vi "Hot Goal Recognition.vi"() -> (0 "Right Goal Hot?":bool, 1 "Left Goal hot?":bool)   [LabVIEW 2013]
uses:
  <vilib>/Rock Robotics/WPI/Camera/WPI_CameraSettings Read MJPG.ctl
  <vilib>/Rock Robotics/WPI/Camera/WPI_CameraImageSize.ctl
  <vilib>/vision/NI_Vision_Development_Module.lvlib
panel:
  out "ERROR":bool
  out "Image":T1(plugin-control)
  out "error out":errorcluster
  in  "Camera IP":string="10.9.0.11"
  out "Bandwidth (Mbps)":dbl
  in  "Camera Settings":T2={"fps"=30, "compression"=30, "Image Size"=enum."320x240"}
  # "do not change resolution!!!! (320x240)"
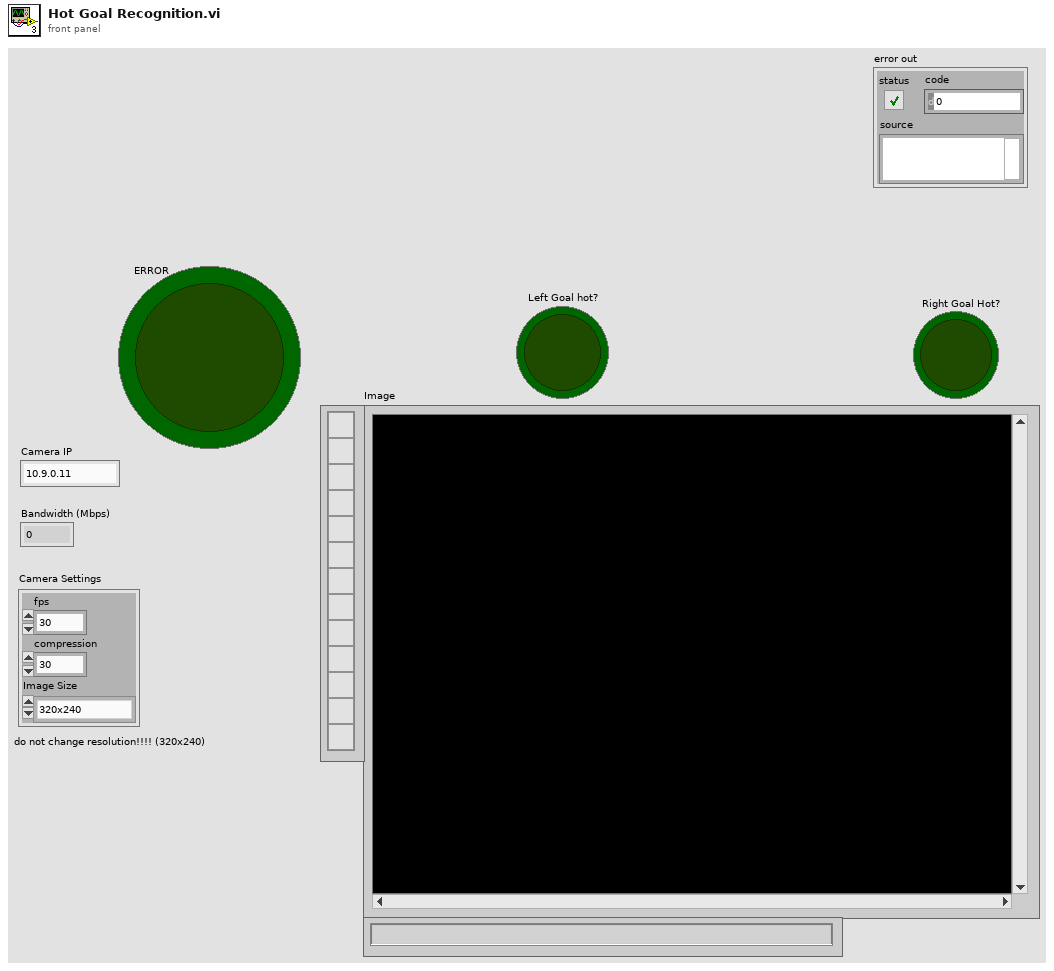
[diagram p1: front panel]
types:
  T1 = typedef "IMAQ Image.ctl" = refnum<image>
  T2 = typedef "WPI_CameraSettings Read MJPG.ctl" = cluster{"fps":i32, "compression":i32, "Image Size":T3}
  T3 = typedef "WPI_CameraImageSize.ctl" = enum16{"640x480", "320x240", "160x120"}
  T4 = typedef "Image Type" = u32
  T5 = enum32{"AutoM", "Close", "Dilate", "Erode", "Gradient", "Gradient in", "Gradient out", "HitMiss", "Open", "PClose", "POpen", "Thick", "Thin"}
  T6 = typedef "Particle Parameters" = i32
  T7 = cluster{"Particle Measurements (Pixels)[0]":dbl, "Particle Measurements (Pixels)[1]":dbl}
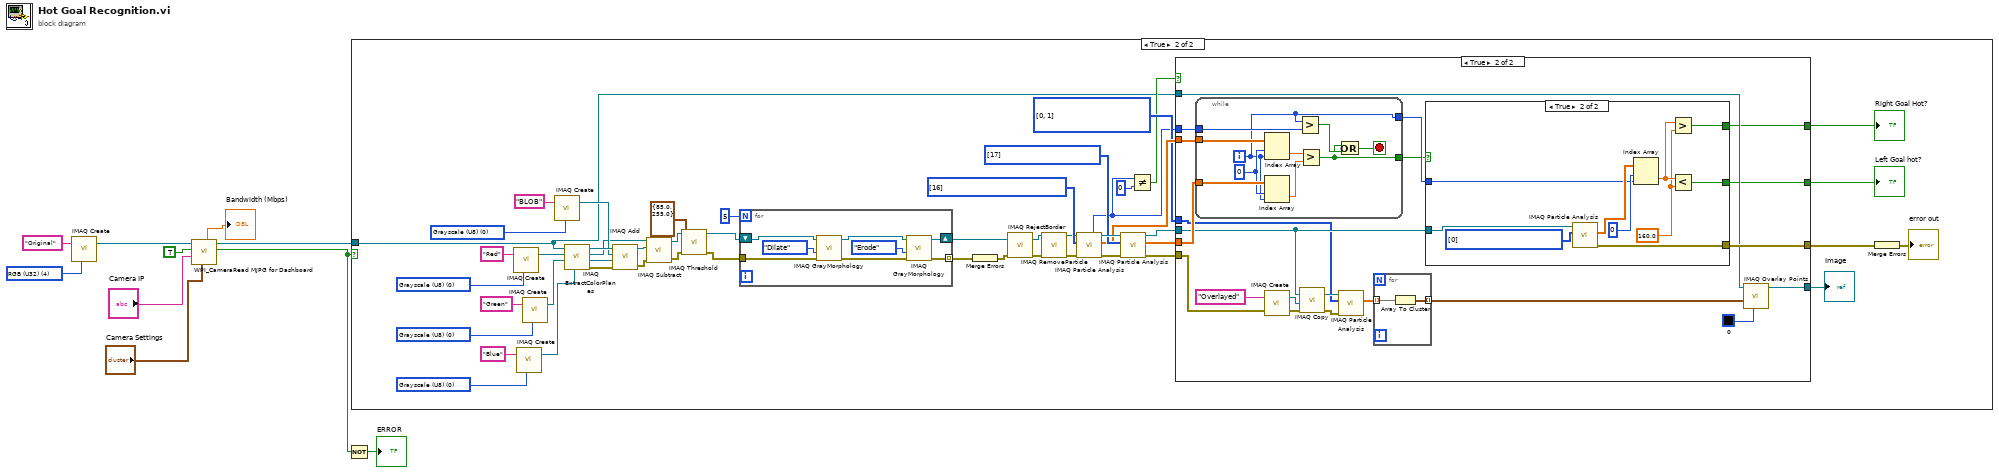
[diagram p0: block diagram]
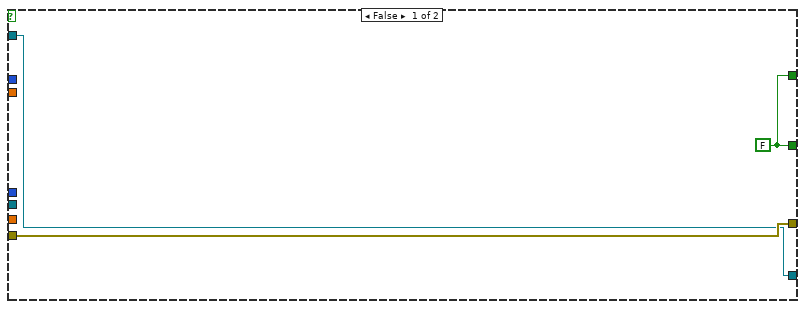
[diagram p3: hidden frame]
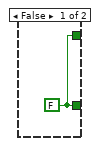
[diagram p4: hidden frame]
diagram:
  w1 = T4 4 items=["Grayscale (U8)", "Grayscale (I16)", "Grayscale (SGL)", "Complex (CSG)", "RGB (U32)", "HSL (U32)", "RGB (U64)", "Grayscale (U16)"] ("Image Type")
  n1 = call "IMAQ Create"("Image Name"="Original", "Image Type"=w1) -> ("New Image"=w9:T1)  [unwired: 3 in, 1 out]
  n2 = call <vilib>:"WPI_CameraRead MJPG for Dashboard.vi"("Camera Settings"="Camera Settings", "Camera IP"="Camera IP", "Enable"=TRUE, "Refnum in"=w9) -> ("Active"=w6:bool, "Refnum out"=w7:T1, "Bandwidth (Mbps)"=→"Bandwidth (Mbps)":dbl)  [unwired: 4 in, 1 out]
  n3 = Not(x=w6) -> (.not. x?=→"ERROR":bool)
  n4 = case shown="True" w6 {
    tunnel: w7 -> [_ w21]
    frame False {
    }
    frame True {
      w26 = T6[] [0, 1] items=["Center of Mass X", "Center of Mass Y", "First Pixel X", "First Pixel Y", "Bounding Rect Left", "Bounding Rect Top", "Bounding Rect Right", "Bounding Rect Bottom", "Max Feret Diameter Start X", "Max Feret Diameter Start Y", "Max Feret Diameter End X", "Max Feret Diameter End Y", "Max Horiz. Segment Length Left", "Max Horiz. Segment Length Right", "Max Horiz. Segment Length Row", "-", "Bounding Rect Width", "Bounding Rect Height", "Bounding Rect Diagonal", "Perimeter", "Convex Hull Perimeter", "Holes' Perimeter", "Max Feret Diameter", "Equivalent Ellipse Major Axis", "Equivalent Ellipse Minor Axis", "Equivalent Ellipse Minor Axis (Feret)", "Equivalent Rect Long Side", "Equivalent Rect Short Side", "Equivalent Rect Diagonal", "Equivalent Rect Short Side (Feret)", "Average Horiz. Segment Length", "Average Vert. Segment Length", "Hydraulic Radius", "Waddel Disk Diameter", "-", "Area", "Holes' Area", "Particle & Holes' Area", "Convex Hull Area", "Image Area", "-", "Number of Holes", "Number of Horiz. Segments", "Number of Vert. Segments", "-", "Orientation", "Max Feret Diameter Orientation", "-", "% Area/Image Area", "% Area/(Particle & Holes' Area)", "Ratio of Equivalent Ellipse Axes", "Ratio of Equivalent Rect Sides", "-", "Elongation Factor", "Compactness Factor", "Heywood Circularity Factor", "Type Factor", "-", "Sum X", "Sum Y", "Sum XX", "Sum XY", "Sum YY", "Sum XXX", "Sum XXY", "Sum XYY", "Sum YYY", "-", "Moment of Inertia XX", "Moment of Inertia XY", "Moment of Inertia YY", "Moment of Inertia XXX", "Moment of Inertia XXY", "Moment of Inertia XYY", "Moment of Inertia YYY", "Norm. Moment of Inertia XX", "Norm. Moment of Inertia XY", "Norm. Moment of Inertia YY", "Norm. Moment of Inertia XXX", "Norm. Moment of Inertia XXY", "Norm. Moment of Inertia XYY", "Norm. Moment of Inertia YYY", "Hu Moment 1", "Hu Moment 2", "Hu Moment 3", "Hu Moment 4", "Hu Moment 5", "Hu Moment 6", "Hu Moment 7"] ("Pixel Measurements")
      w45 = T4 0 items=["Grayscale (U8)", "Grayscale (I16)", "Grayscale (SGL)", "Complex (CSG)", "RGB (U32)", "HSL (U32)", "RGB (U64)", "Grayscale (U16)"] ("Image Type")
      w48 = T4 0 items=["Grayscale (U8)", "Grayscale (I16)", "Grayscale (SGL)", "Complex (CSG)", "RGB (U32)", "HSL (U32)", "RGB (U64)", "Grayscale (U16)"] ("Image Type")
      w50 = T4 0 items=["Grayscale (U8)", "Grayscale (I16)", "Grayscale (SGL)", "Complex (CSG)", "RGB (U32)", "HSL (U32)", "RGB (U64)", "Grayscale (U16)"] ("Image Type")
      w55 = T6[] [17] items=["Center of Mass X", "Center of Mass Y", "First Pixel X", "First Pixel Y", "Bounding Rect Left", "Bounding Rect Top", "Bounding Rect Right", "Bounding Rect Bottom", "Max Feret Diameter Start X", "Max Feret Diameter Start Y", "Max Feret Diameter End X", "Max Feret Diameter End Y", "Max Horiz. Segment Length Left", "Max Horiz. Segment Length Right", "Max Horiz. Segment Length Row", "-", "Bounding Rect Width", "Bounding Rect Height", "Bounding Rect Diagonal", "Perimeter", "Convex Hull Perimeter", "Holes' Perimeter", "Max Feret Diameter", "Equivalent Ellipse Major Axis", "Equivalent Ellipse Minor Axis", "Equivalent Ellipse Minor Axis (Feret)", "Equivalent Rect Long Side", "Equivalent Rect Short Side", "Equivalent Rect Diagonal", "Equivalent Rect Short Side (Feret)", "Average Horiz. Segment Length", "Average Vert. Segment Length", "Hydraulic Radius", "Waddel Disk Diameter", "-", "Area", "Holes' Area", "Particle & Holes' Area", "Convex Hull Area", "Image Area", "-", "Number of Holes", "Number of Horiz. Segments", "Number of Vert. Segments", "-", "Orientation", "Max Feret Diameter Orientation", "-", "% Area/Image Area", "% Area/(Particle & Holes' Area)", "Ratio of Equivalent Ellipse Axes", "Ratio of Equivalent Rect Sides", "-", "Elongation Factor", "Compactness Factor", "Heywood Circularity Factor", "Type Factor", "-", "Sum X", "Sum Y", "Sum XX", "Sum XY", "Sum YY", "Sum XXX", "Sum XXY", "Sum XYY", "Sum YYY", "-", "Moment of Inertia XX", "Moment of Inertia XY", "Moment of Inertia YY", "Moment of Inertia XXX", "Moment of Inertia XXY", "Moment of Inertia XYY", "Moment of Inertia YYY", "Norm. Moment of Inertia XX", "Norm. Moment of Inertia XY", "Norm. Moment of Inertia YY", "Norm. Moment of Inertia XXX", "Norm. Moment of Inertia XXY", "Norm. Moment of Inertia XYY", "Norm. Moment of Inertia YYY", "Hu Moment 1", "Hu Moment 2", "Hu Moment 3", "Hu Moment 4", "Hu Moment 5", "Hu Moment 6", "Hu Moment 7"] ("Pixel Measurements")
      w57 = T6[] [16] items=["Center of Mass X", "Center of Mass Y", "First Pixel X", "First Pixel Y", "Bounding Rect Left", "Bounding Rect Top", "Bounding Rect Right", "Bounding Rect Bottom", "Max Feret Diameter Start X", "Max Feret Diameter Start Y", "Max Feret Diameter End X", "Max Feret Diameter End Y", "Max Horiz. Segment Length Left", "Max Horiz. Segment Length Right", "Max Horiz. Segment Length Row", "-", "Bounding Rect Width", "Bounding Rect Height", "Bounding Rect Diagonal", "Perimeter", "Convex Hull Perimeter", "Holes' Perimeter", "Max Feret Diameter", "Equivalent Ellipse Major Axis", "Equivalent Ellipse Minor Axis", "Equivalent Ellipse Minor Axis (Feret)", "Equivalent Rect Long Side", "Equivalent Rect Short Side", "Equivalent Rect Diagonal", "Equivalent Rect Short Side (Feret)", "Average Horiz. Segment Length", "Average Vert. Segment Length", "Hydraulic Radius", "Waddel Disk Diameter", "-", "Area", "Holes' Area", "Particle & Holes' Area", "Convex Hull Area", "Image Area", "-", "Number of Holes", "Number of Horiz. Segments", "Number of Vert. Segments", "-", "Orientation", "Max Feret Diameter Orientation", "-", "% Area/Image Area", "% Area/(Particle & Holes' Area)", "Ratio of Equivalent Ellipse Axes", "Ratio of Equivalent Rect Sides", "-", "Elongation Factor", "Compactness Factor", "Heywood Circularity Factor", "Type Factor", "-", "Sum X", "Sum Y", "Sum XX", "Sum XY", "Sum YY", "Sum XXX", "Sum XXY", "Sum XYY", "Sum YYY", "-", "Moment of Inertia XX", "Moment of Inertia XY", "Moment of Inertia YY", "Moment of Inertia XXX", "Moment of Inertia XXY", "Moment of Inertia XYY", "Moment of Inertia YYY", "Norm. Moment of Inertia XX", "Norm. Moment of Inertia XY", "Norm. Moment of Inertia YY", "Norm. Moment of Inertia XXX", "Norm. Moment of Inertia XXY", "Norm. Moment of Inertia XYY", "Norm. Moment of Inertia YYY", "Hu Moment 1", "Hu Moment 2", "Hu Moment 3", "Hu Moment 4", "Hu Moment 5", "Hu Moment 6", "Hu Moment 7"] ("Pixel Measurements")
      w58 = T4 0 items=["Grayscale (U8)", "Grayscale (I16)", "Grayscale (SGL)", "Complex (CSG)", "RGB (U32)", "HSL (U32)", "RGB (U64)", "Grayscale (U16)"] ("Image Type")
      n5 = call "IMAQ Create"("Image Name"="Red", "Image Type"=w50) -> ("New Image"=w51:T1)  [unwired: 3 in, 1 out]
      n6 = call "IMAQ Create"("Image Name"="Blue", "Image Type"=w45) -> ("New Image"=w44:T1)  [unwired: 3 in, 1 out]
      n7 = call "IMAQ Create"("Image Name"="Green", "Image Type"=w48) -> ("New Image"=w47:T1)  [unwired: 3 in, 1 out]
      n8 = call "IMAQ Create"("Image Name"="BLOB", "Image Type"=w58) -> ("New Image"=w41:T1)  [unwired: 3 in, 1 out]
      n9 = call "IMAQ ExtractColorPlanes"("Blue or Luma or Val or Inten Plane"=w44, "Green or Sat Plane"=w47, "Red or Hue Plane"=w51, "Image Src"=w21) -> ("error out"=w18:errorcluster, "Blue or Luma or Val or Inten Plane out"=w42:T1, "Green or Sat Plane out"=w40:T1, "Red or Hue Plane out"=w43:T1)  [unwired: 4 in]
      n10 = call "IMAQ Add"("Image Src A"=w43, "Image Dst"=w41, "Image Src B"=w42, "error in (no error)"=w18) -> ("Image Dst Out"=w17:T1, "error out"=w14:errorcluster)  [unwired: 3 in]
      n11 = call "IMAQ Subtract"("Image Src A"=w40, "Image Dst"=w17, "error in (no error)"=w14) -> ("Image Dst Out"=w15:T1, "error out"=w13:errorcluster)  [unwired: 4 in]
      n12 = call "IMAQ Threshold"("error in (no error)"=w13, "Range"=cluster{"Lower value":sgl, "Upper value":sgl} {"Lower value"=85.0, "Upper value"=255.0}, "Image Src"=w15) -> ("error out"=w12:errorcluster, "Image Dst Out"=w16:T1)  [unwired: 7 in]
      n13 = for {
        N: 5 -> [_]
        shift-right: [w110] -> w38
        shift-left: w16 -> [w111]
        tunnel: w12 -> [w109]
        tunnel: [w107] -> w35 mode=indexing
        n14 = call "IMAQ GrayMorphology"("error in (no error)"=w109, "Operation"=T5."Dilate", "Image Src"=w111) -> ("error out"=w108:errorcluster, "Image Dst Out"=w112:T1)  [unwired: 7 in]
        n15 = call "IMAQ GrayMorphology"("error in (no error)"=w108, "Operation"=T5."Erode", "Image Src"=w112) -> ("error out"=w107:errorcluster, "Image Dst Out"=w110:T1)  [unwired: 7 in]
      }
      n16 = Merge Errors(w35) -> (w34:errorcluster)
      n17 = call "IMAQ RejectBorder"("error in (no error)"=w34, "Image Src"=w38) -> ("error out"=w36:errorcluster, "Image Dst Out"=w37:T1)  [unwired: 4 in]
      n18 = call "IMAQ RemoveParticle"("error in (no error)"=w36, "Image Src"=w37) -> ("error out"=w29:errorcluster, "Image Dst Out"=w30:T1)  [unwired: 8 in]
      n19 = call "IMAQ Particle Analysis"("error in (no error)"=w29, "Pixel Measurements"=w57, "Image"=w30) -> ("error out"=w33:errorcluster, "Particle Measurements (Pixels)"=w54:dbl[][], "Image Out (duplicate)"=w56:T1, "Number of Particles"=w25:i32)  [unwired: 3 in, 2 out]
      n20 = call "IMAQ Particle Analysis"("error in (no error)"=w33, "Pixel Measurements"=w55, "Image"=w56) -> ("error out"=w27:errorcluster, "Particle Measurements (Pixels)"=w53:dbl[][], "Image Out (duplicate)"=w28:T1)  [unwired: 3 in, 3 out]
      n21 = Not Equal?(x=w25, y=0) -> (x != y?=w23:bool)
      n22 = case shown="True" w23 {
        tunnel: w54 -> [_ w83]
        tunnel: w53 -> [_ w82]
        tunnel: w25 -> [_ w81]
        tunnel: [w62 w78] -> w32
        tunnel: w28 -> [_ w75]
        tunnel: w27 -> [w62 w74]
        tunnel: w26 -> [_ w70]
        tunnel: [w61 w66] -> w22
        tunnel: w21 -> [w61 w65]
        tunnel: [w60 w64] -> w20
        tunnel: [w60 w63] -> w19
        frame False {
          w60 = FALSE
        }
        frame True {
          n23 = while {
            tunnel: w83 -> [w105]
            tunnel: w82 -> [w106]
            tunnel: w81 -> [w99]
            tunnel: [w98] -> w79
            tunnel: [w97] -> w80
            i -> [w97]
            stop <- w100 stop-if-true
            w104 = 0 ("disabled index (row)")
            n24 = Index Array(array=w105, index (row)=w104, index (col)=w97) -> (element=w102:dbl)
            n25 = Index Array(array=w106, index (row)=w104, index (col)=w97) -> (element=w103:dbl)
            n26 = Greater?(x=w97, y=w99) -> (0:w101:bool)
            n27 = Greater?(x=w102, y=w103) -> (0:w98:bool)
            n28 = Or(x=w98, y=w101) -> (x .or. y?=w100:bool)
          }
          n29 = call "IMAQ Create"("Image Name"="Overlayed", "error in (no error)"=w74) -> ("New Image"=w76:T1, "error out"=w73:errorcluster)  [unwired: 3 in]
          n30 = call "IMAQ Copy"("error in (no error)"=w73, "Image Dst"=w76, "Image Src"=w75) -> ("error out"=w72:errorcluster, "Image Dst Out"=w71:T1)  [unwired: 3 in]
          n31 = call "IMAQ Particle Analysis"("error in (no error)"=w72, "Pixel Measurements"=w70, "Image"=w71) -> ("Particle Measurements (Pixels)"=w67:dbl[][])  [unwired: 3 in, 5 out]
          n32 = for {
            tunnel: w67 -> [w85] mode=indexing
            tunnel: [w84] -> w68 mode=indexing
            n33 = Array To Cluster(array=w85) -> (cluster=w84:T7)
          }
          n34 = case shown="True" w79 {
            tunnel: w80 -> [_ w92]
            tunnel: w75 -> [_ w95]
            tunnel: [_ w91] -> w78
            tunnel: [w86 w88] -> w64
            tunnel: [w86 w87] -> w63
            frame False {
              w86 = FALSE
            }
            frame True {
              w89 = 160.0 ("y")
              w96 = T6[] [0] items=["Center of Mass X", "Center of Mass Y", "First Pixel X", "First Pixel Y", "Bounding Rect Left", "Bounding Rect Top", "Bounding Rect Right", "Bounding Rect Bottom", "Max Feret Diameter Start X", "Max Feret Diameter Start Y", "Max Feret Diameter End X", "Max Feret Diameter End Y", "Max Horiz. Segment Length Left", "Max Horiz. Segment Length Right", "Max Horiz. Segment Length Row", "-", "Bounding Rect Width", "Bounding Rect Height", "Bounding Rect Diagonal", "Perimeter", "Convex Hull Perimeter", "Holes' Perimeter", "Max Feret Diameter", "Equivalent Ellipse Major Axis", "Equivalent Ellipse Minor Axis", "Equivalent Ellipse Minor Axis (Feret)", "Equivalent Rect Long Side", "Equivalent Rect Short Side", "Equivalent Rect Diagonal", "Equivalent Rect Short Side (Feret)", "Average Horiz. Segment Length", "Average Vert. Segment Length", "Hydraulic Radius", "Waddel Disk Diameter", "-", "Area", "Holes' Area", "Particle & Holes' Area", "Convex Hull Area", "Image Area", "-", "Number of Holes", "Number of Horiz. Segments", "Number of Vert. Segments", "-", "Orientation", "Max Feret Diameter Orientation", "-", "% Area/Image Area", "% Area/(Particle & Holes' Area)", "Ratio of Equivalent Ellipse Axes", "Ratio of Equivalent Rect Sides", "-", "Elongation Factor", "Compactness Factor", "Heywood Circularity Factor", "Type Factor", "-", "Sum X", "Sum Y", "Sum XX", "Sum XY", "Sum YY", "Sum XXX", "Sum XXY", "Sum XYY", "Sum YYY", "-", "Moment of Inertia XX", "Moment of Inertia XY", "Moment of Inertia YY", "Moment of Inertia XXX", "Moment of Inertia XXY", "Moment of Inertia XYY", "Moment of Inertia YYY", "Norm. Moment of Inertia XX", "Norm. Moment of Inertia XY", "Norm. Moment of Inertia YY", "Norm. Moment of Inertia XXX", "Norm. Moment of Inertia XXY", "Norm. Moment of Inertia XYY", "Norm. Moment of Inertia YYY", "Hu Moment 1", "Hu Moment 2", "Hu Moment 3", "Hu Moment 4", "Hu Moment 5", "Hu Moment 6", "Hu Moment 7"] ("Pixel Measurements")
              n35 = call "IMAQ Particle Analysis"("Pixel Measurements"=w96, "Image"=w95) -> ("error out"=w91:errorcluster, "Particle Measurements (Pixels)"=w94:dbl[][])  [unwired: 4 in, 4 out]
              n36 = Index Array(array=w94, index (row)=0, index (col)=w92) -> (element=w90:dbl)
              n37 = Greater?(x=w90, y=w89) -> (0:w88:bool)
              n38 = Less?(x=w90, y=w89) -> (x < y?=w87:bool)
            }
          }
          n39 = call "IMAQ Overlay Points"("Color"=u32 0, "Array of Points"=w68, "Image"=w65) -> ("Image Out"=w66:T1)  [unwired: 7 in, 1 out]
        }
      }
      "Image" <- w22
      "Right Goal Hot?" <- w20
      "Left Goal hot?" <- w19
      n40 = Merge Errors(w32) -> (→"error out":errorcluster)
    }
  }
